vi "Check_Execution_Row.vi"(0 "Execution Row":T1 {"Row Duration (mins)" format="%#.1f"; "Row No" min=0; "Trace Gas Concentration (%)" min=0.0 format="%#.2f"; "Emission Rate (l/min)" format="%#.2f"; "Tunnel Speed" format="%#.2f"; "Start X" format="%#.2f"; "Start Y" format="%#.2f"; "Start Z" format="%#.2f"; "End X" format="%#.2f"; "End Y" format="%#.2f"; "End Z" format="%#.2f"; "Averaging time (min)" min=0.0 format="%#.2f"}, 3 "Synchronization Start No":i32=1 min=1 max=100, 4 "Row Index":i32, 5 "Max Tunnel Speed":dbl format="%.2f") -> (6 "Editted Row":bool, 7 "Execution Row Out":T1 {"Row Duration (mins)" format="%#.1f"; "Row No" min=0; "Trace Gas Concentration (%)" min=0.0 format="%#.2f"; "Emission Rate (l/min)" format="%#.2f"; "Tunnel Speed" format="%#.2f"; "Start X" format="%#.2f"; "Start Y" format="%#.2f"; "Start Z" format="%#.2f"; "End X" format="%#.2f"; "End Y" format="%#.2f"; "End Z" format="%#.2f"; "Averaging time (min)" min=0.0 format="%#.2f"}, 9 "Continue?":bool, 10 "Error Comments":string)   [LabVIEW 2012]
uses:
  Traverse_cluster.ctl
  Spacing.ctl
  Controls/Multi_run_mode.ctl
  Controls/User_Specific_mode.ctl
  Controls/Tunnel_Coordinates.ctl
  ADAM Client/Sub VIs/ADAM Controls/Channel_names.ctl
  Globals/Extra_Commands_Global.vi
  Globals/Constants_global.vi
  Globals/Trav_pos_global.vi
panel:
  out "Traverse line Out":T1 {"Row Duration (mins)" format="%#.1f"; "Row No" min=0; "Trace Gas Concentration (%)" min=0.0 format="%#.2f"; "Emission Rate (l/min)" format="%#.2f"; "Tunnel Speed" format="%#.2f"; "Start X" format="%#.2f"; "Start Y" format="%#.2f"; "Start Z" format="%#.2f"; "End X" format="%#.2f"; "End Y" format="%#.2f"; "End Z" format="%#.2f"; "Averaging time (min)" min=0.0 format="%#.2f"}
  out "Fixed Axis":bool[](array[boolean])
  out "Filenames":string[](array[string])
  out "Current Sync Number":i32
  out "Checks":string[](array[string])
  in  "Edit in Excel":bool
  in  "OK":bool
  # "X           Y            Z"
  # "Start"
  # "End"
  # "X           Y            Z"
  # "Start"
  # "End"
  # "X           Y            Z"
  # "Start"
  # "End"
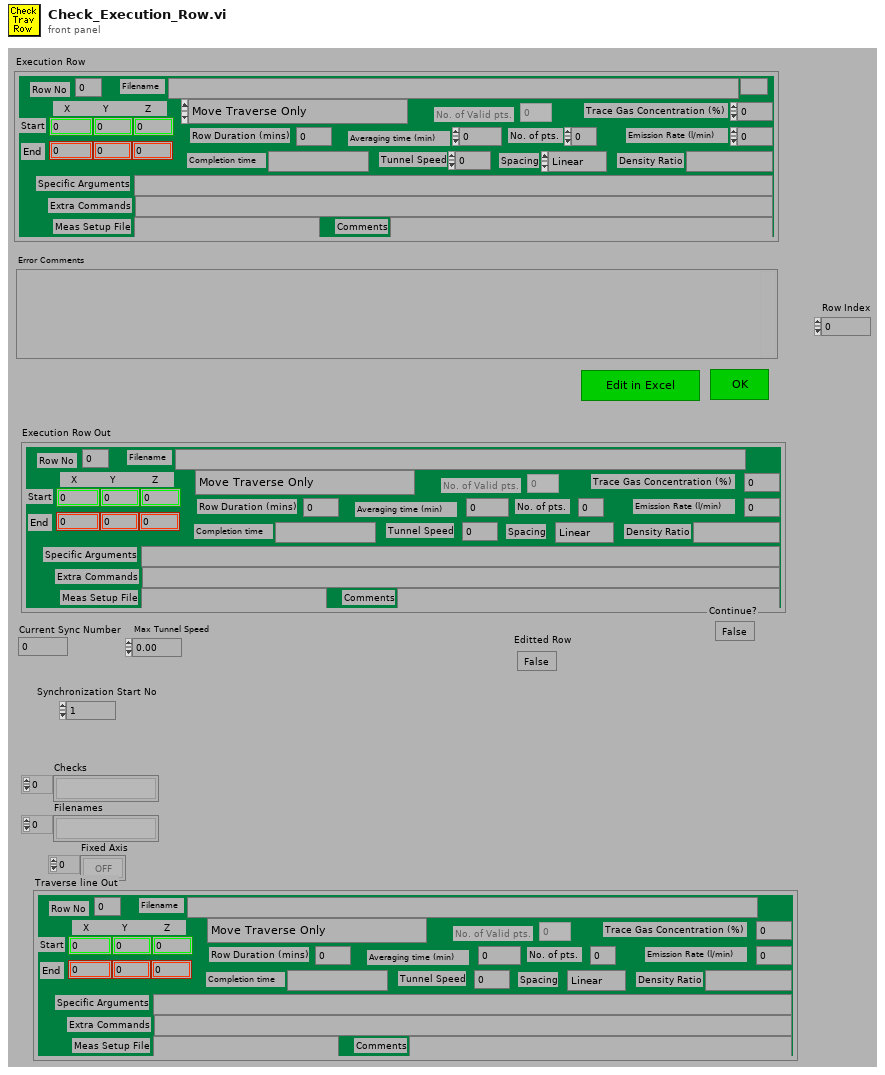
[diagram p1: front panel]
types:
  T1 = typedef "Traverse_cluster.ctl" = cluster{"Start X":dbl, "Start Y":dbl, "Start Z":dbl, "End X":dbl, "End Y":dbl, "End Z":dbl, "No. of pts.":i32, "Spacing":T2, "Filename":path, "Tunnel Speed":dbl, "Averaging time (min)":dbl, "Extra Commands":string, "Specific Arguments":string, "Emission Rate (l/min)":dbl, "Trace Gas Concentration (%)":dbl, "Density Ratio":string, "Comments":string, "Row No":i32, "Row Type Selector":T3, "Completion time":string, "Row Duration (mins)":dbl, "No. of Valid pts.":i32, "Meas Setup File":string}
  T2 = typedef "Spacing.ctl" = enum16{"Linear", "Log", "Gauss", "Specified", "N/A"}
  T3 = typedef "Multi_run_mode.ctl" = enum16{"Move Traverse Only", "Set Tunnel Speed Only", "Set Source Only", "Set Measurement Conditions", "Single Measurement", "Vertical Profile", "Lateral Profile", "Longitudinal Profile", "Explore Volume", "Multi-Axis Profile", "Auto Calibrate", "Meas Fast FID Bkgnd", "Check Beam Power", "Scanning Valve Measurement", "Run VI Named:", "Set ADAM Ch", "Wait (minutes)", "Send Message", "Synchronize With:", "Fall Back to this Row", "Turn Off Row Repeating", "Blank Row", "Traverse 3D Volume"}
  T4 = enum16{"All Channel Names", "Valid Channel Names"}
  T5 = typedef "User_Specific_mode.ctl" = enum16{"Check VI only", "Run VI"}
  T6 = typedef "Tunnel_Coordinates.ctl" = enum16{"Work in Tunnel Coordinates", "Work in Model Coordinates"}
  T7 = enum16{"Zero or one", "One", "Zero or more", "One or more"}
  T8 = typedef "Channel_names.ctl" = enum16{"Active Only", "Active + Off", "All Channels"}
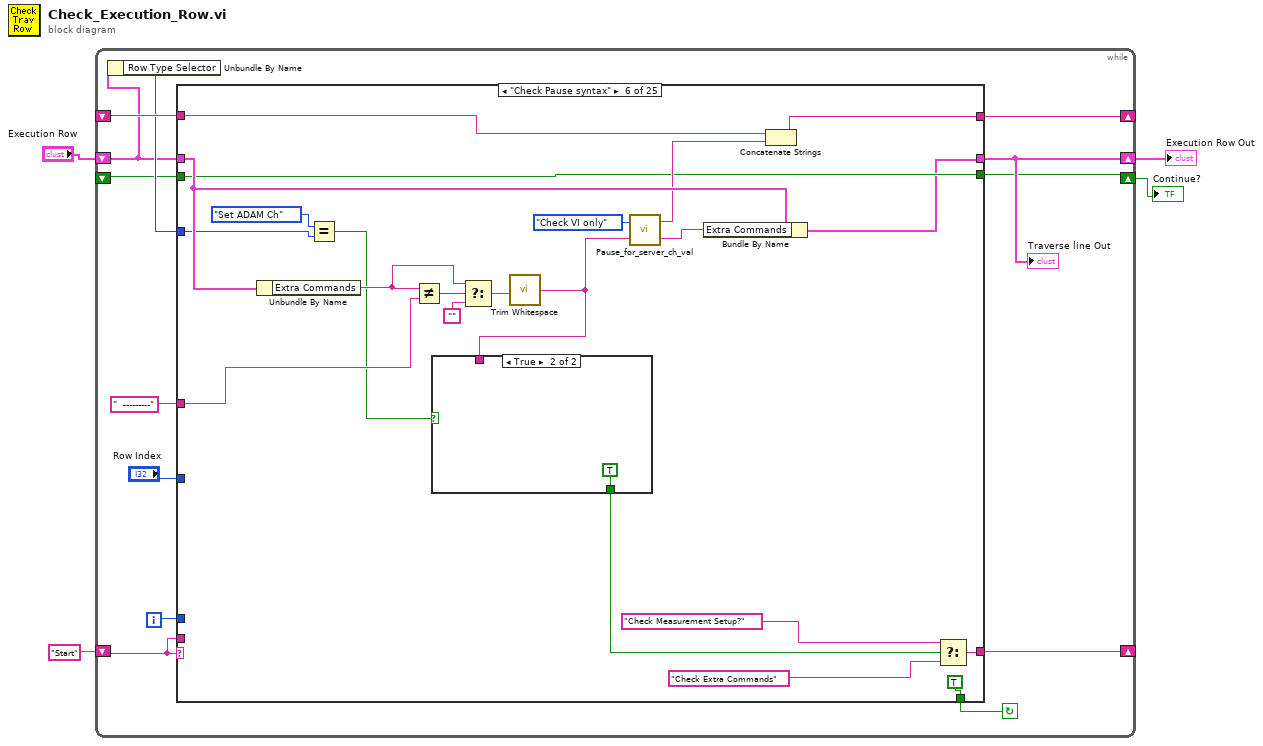
[diagram p0: block diagram]
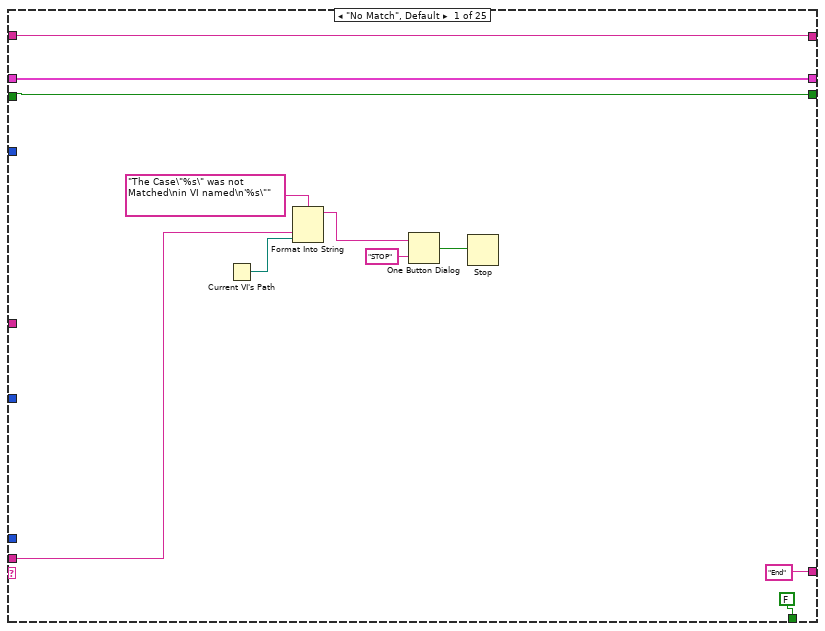
[diagram p2: hidden frame]
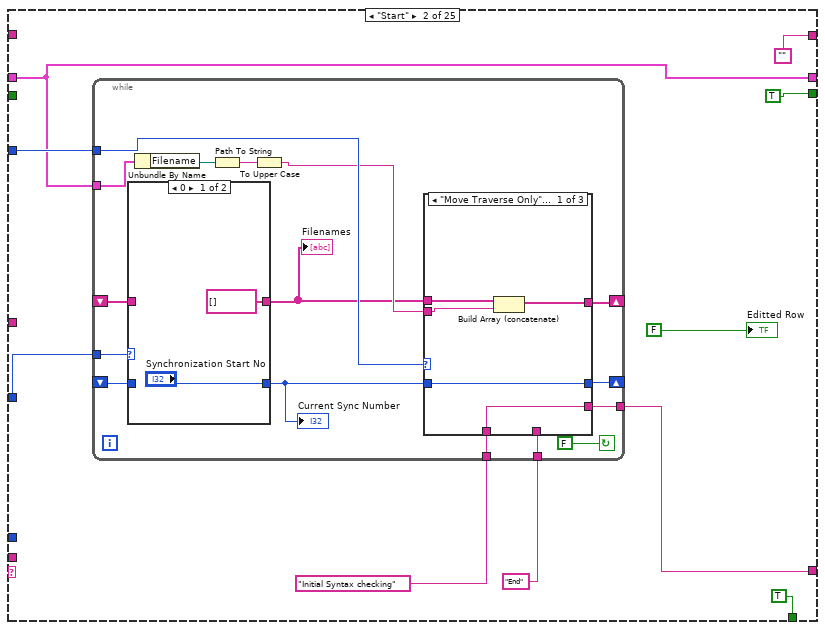
[diagram p3: hidden frame]
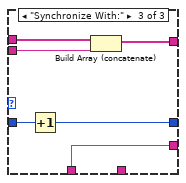
[diagram p6: hidden frame]
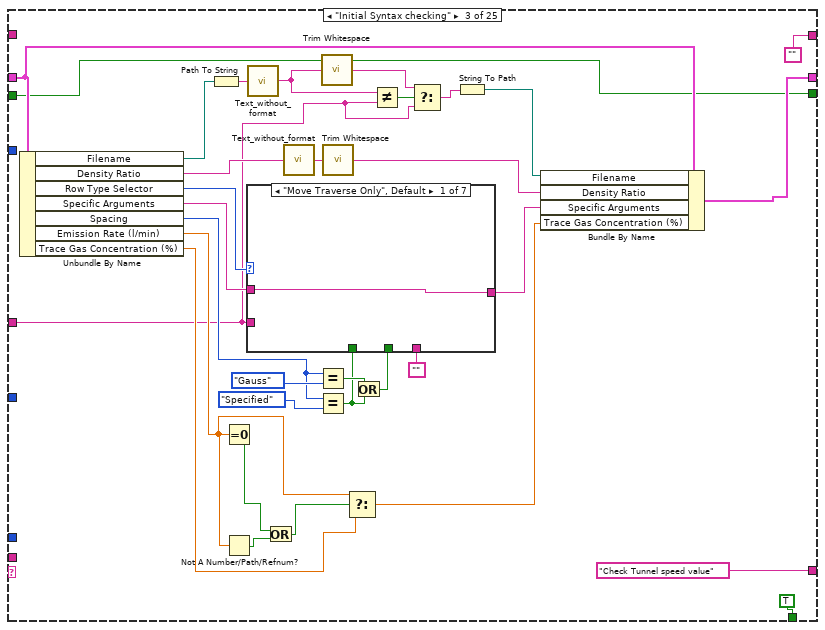
[diagram p7: hidden frame]
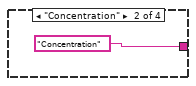
[diagram p9: hidden frame]
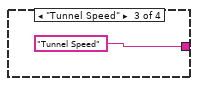
[diagram p10: hidden frame]
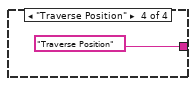
[diagram p11: hidden frame]
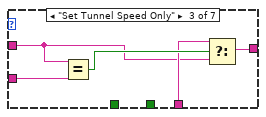
[diagram p12: hidden frame]
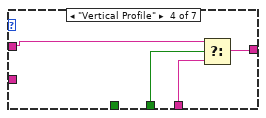
[diagram p13: hidden frame]
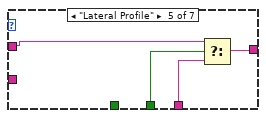
[diagram p14: hidden frame]
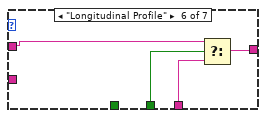
[diagram p15: hidden frame]
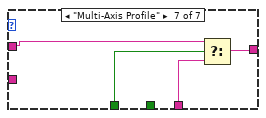
[diagram p16: hidden frame]
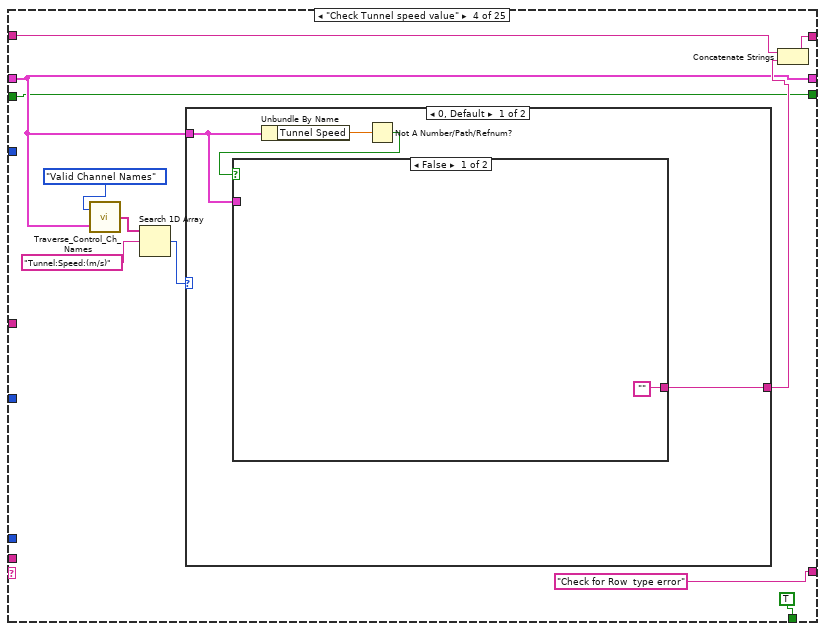
[diagram p17: hidden frame]
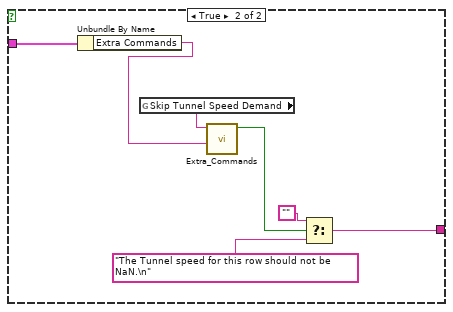
[diagram p18: hidden frame]
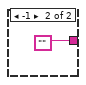
[diagram p19: hidden frame]
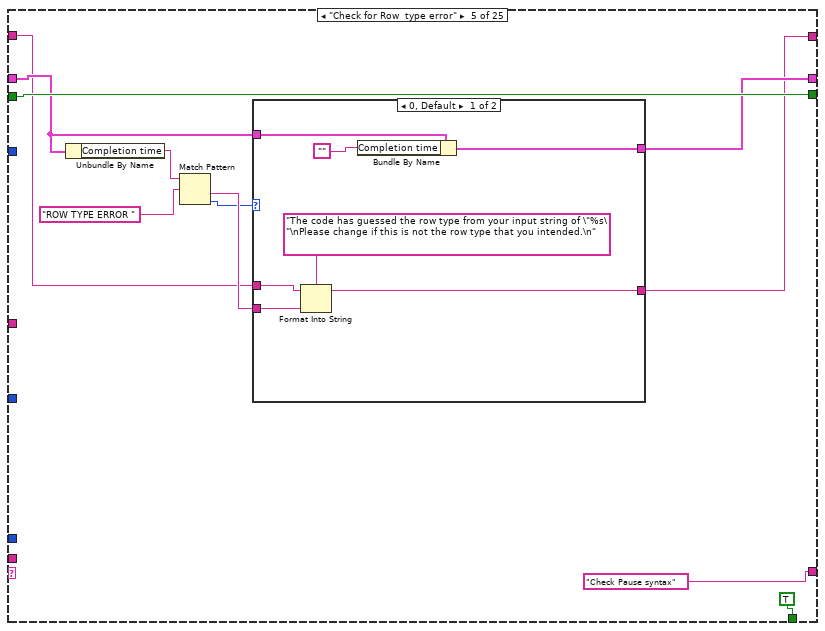
[diagram p20: hidden frame]
diagram:
  n1 = while {
    shift-left: _ -> [w16]
    shift-right: [w17] -> _
    shift-left: "Start" -> [w9]
    shift-right: [w14] -> _
    shift-right: [w8] -> w2
    shift-left: "Execution Row" -> [w5]
    shift-right: [w7] -> w1
    shift-left: _ -> [w6]
    i -> [w10]
    stop <- w15 continue-if-true
    n2 = Unbundle By Name(w5) -> ("Row Type Selector"=w12:T3)
    n3 = case shown="\"Check Pause syntax\"" w9 {
      tunnel: w5 -> [w22 w32 w100 w137 w161 w193 w211 w252 w282 w338 w371 w379 w418 w762 w862 w899 w927 w1012 w1044 w1054 w1123 _ w1162 w1169 w1179]
      tunnel: "  ---------" ("f") -> [_ _ w74 _ _ w197 _ _ _ _ _ _ _ _ _ _ _ _ _ _ _ _ _ _ _]
      tunnel: "Row Index" -> [_ w36 _ _ _ _ w208 _ _ _ _ _ w412 _ _ _ _ _ _ _ _ _ w1163 _ w1178]
      tunnel: [w21 "" "" w138 w158 w186 w219 w257 w287 w340 w375 w384 w422 w767 w872 w905 w950 w1010 w1048 w1055 w1129 w1140 w1164 w1174 w1181] -> w17
      tunnel: w12 -> [_ w35 _ _ _ w179 _ _ _ _ _ w382 w421 w763 w860 _ _ _ _ w1059 _ _ _ _ _]
      tunnel: w16 -> [w21 _ _ w139 w159 w188 w220 w258 w288 w340 w374 w385 w423 w767 w873 w906 w951 w1010 w1049 w1060 w1129 w1140 w1164 w1174 w1181]
      tunnel: [FALSE TRUE TRUE TRUE TRUE TRUE TRUE TRUE TRUE TRUE TRUE TRUE TRUE TRUE TRUE TRUE TRUE TRUE TRUE w1051 TRUE TRUE TRUE TRUE FALSE] -> w15
      tunnel: ["End" w33 "Check Tunnel speed value" ("f") "Check for Row  type error" ("f") "Check Pause syntax" ("f") w191 "Check Traverse Setup Name" ("f") "Check IF command" ("f") "Check Measurement Setup?" ("f") w342 "Check Maximum tunnel speed" ("f") "Row type specific check" ("f") w419 "Check for position NaNs" ("f") w863 "Check source details" ("t") "Check source details" ("f") w1007 "check entered filename etc" ("f") w1057 "What to do next?" ("f") w1138 "Initial Syntax checking" "End" "End"] -> w14
      tunnel: w10 -> [_ _ _ _ _ _ _ _ _ _ _ _ _ _ _ _ _ _ _ _ _ _ _ _ _]
      tunnel: w9 -> [w23 _ _ _ _ _ _ _ _ _ _ _ _ _ _ _ _ _ _ _ _ _ _ _ _]
      tunnel: [w22 w32 w77 w137 w162 w181 w210 w252 w282 w338 w370 w379 w413 w761 w862 w899 w926 w1011 w1044 w1053 w1123 w1131 w1165 w1169 w1177] -> w8
      tunnel: [w18 TRUE w75 w136 w168 w182 w212 w249 w279 w344 w372 w377 w415 w759 w861 w898 w924 w1015 w1042 w1051 w1122 w1130 w1159 w1168 w1175] -> w7
      tunnel: w6 -> [w18 _ w75 w136 w168 w182 w212 w249 w279 w344 w372 w377 w415 w759 w861 w898 w924 w1015 w1042 _ w1122 _ w1159 w1168 w1175]
      frame "No Match", Default {
        n4 = Current VI's Path() -> (path=w24:path)
        n5 = Format Into String(format string="The Case\"%s\" was not Matched\nin VI named\n'%s\"" ("Format String"), w23, w24) -> (resulting string=w27:string)  [unwired: 2 in, 1 out]
        n6 = One Button Dialog(message=w27, button name ("OK")="STOP") -> (true=w25:bool)
        n7 = Stop(stop? (T)=w25) -> ()
      }
      frame "Start" {
        n8 = while {
          tunnel: "End" -> [w40]
          tunnel: "Initial Syntax checking" -> [w41]
          tunnel: [w42] -> w33
          tunnel: w32 -> [w49]
          shift-left: _ -> [w48]
          shift-right: [w47] -> _
          tunnel: w35 -> [w53]
          shift-left: _ -> [w52]
          shift-right: [w51] -> _
          tunnel: w36 -> [w54]
          stop <- FALSE continue-if-true
          n9 = case shown="0" w54 {
            tunnel: ["Synchronization Start No" w58] -> w50
            tunnel: w52 -> [_ w58]
            tunnel: w48 -> [_ w57]
            tunnel: [string[] [] w57] -> w43
            frame 0 {
            }
            frame 1, Default {
            }
          }
          "Current Sync Number" <- w50
          "Filenames" <- w43
          n10 = Unbundle By Name(w49) -> ("Filename"=w46:path)
          n11 = Path To String(path=w46) -> (string=w45:string)
          n12 = To Upper Case(1:w45) -> (0:w44:string)
          n13 = case shown="\"Move Traverse Only\", Default" w53 {
            tunnel: w50 -> [w63 w66 w72]
            tunnel: [w63 w66 w71] -> w51
            tunnel: w44 -> [w61 _ w70]
            tunnel: w43 -> [w62 w65 w69]
            tunnel: [w60 w65 w68] -> w47
            tunnel: [w59 w64 w67] -> w42
            tunnel: w41 -> [w59 _ w67]
            tunnel: w40 -> [_ w64 _]
            frame "Move Traverse Only", Default {
              n14 = Build Array (concatenate)(w62, w61) -> (w60:string[])
            }
            frame "Blank Row" {
            }
            frame "Synchronize With:" {
              n15 = Increment(x=w72) -> (x+1=w71:i32)
              n16 = Build Array (concatenate)(w69, w70) -> (w68:string[])
            }
          }
        }
        "Editted Row" <- FALSE ("Editted Row")
      }
      frame "Initial Syntax checking" {
        n17 = Unbundle By Name(w100) -> ("Filename"=w73:path, "Density Ratio"=w79:string, "Row Type Selector"=w97:T3, "Specific Arguments"=w95:string, "Spacing"=w87:T2, "Emission Rate (l/min)"=w83:dbl, "Trace Gas Concentration (%)"=w93:dbl)
        n18 = Path To String(path=w73) -> (string=w81:string)
        n19 = Equal To 0?(x=w83) -> (x = 0?=w85:bool)
        n20 = Not A Number/Path/Refnum?(number/path/refnum=w83) -> (NaN/Path/Refnum?=w84:bool)
        n21 = call "Text_without_format.vi"("Input string"=w81) -> ("Output string"=w104:string)
        n22 = Or(x=w85, y=w84) -> (x .or. y?=w82:bool)
        n23 = call "Text_without_format.vi"("Input string"=w79) -> ("Output string"=w99:string)
        n24 = Equal?(x=w87, y=Spacing."Gauss" ("Spacing")) -> (x = y?=w89:bool)
        n25 = Equal?(x=w87, y=Spacing."Specified" ("Spacing")) -> (x = y?=w86:bool)
        n26 = call <vilib>:"Trim Whitespace.vi"("string"=w104) -> ("trimmed string"=w103:string)  [unwired: 1 in]
        n27 = call <vilib>:"Trim Whitespace.vi"("string"=w99) -> ("trimmed string"=w78:string)  [unwired: 1 in]
        n28 = Select(t=w83, s=w82, f=w93) -> (s? t:f=w92:dbl)
        n29 = Or(x=w89, y=w86) -> (x .or. y?=w88:bool)
        n30 = case shown="\"Move Traverse Only\", Default" w97 {
          tunnel: [w106 w108 w113 w119 w123 w127 w131] -> w96
          tunnel: w95 -> [w106 w107 w114 w121 w125 w129 w133]
          tunnel: "" -> [_ _ w115 w120 w124 w128 w132]
          tunnel: w88 -> [_ _ _ w118 w122 w126 _]
          tunnel: w86 -> [_ _ _ _ _ _ w130]
          tunnel: w74 -> [_ _ w117 _ _ _ _]
          frame "Move Traverse Only", Default {
          }
          frame "Auto Calibrate" {
            n31 = case shown="\"No Match\", Default" w107 {
              tunnel: [w109 "Concentration" "Tunnel Speed" "Traverse Position"] -> w108
              tunnel: w107 -> [w109 _ _ _]
              frame "No Match", Default {
              }
              frame "Concentration" {
              }
              frame "Tunnel Speed" {
              }
              frame "Traverse Position" {
              }
            }
          }
          frame "Set Tunnel Speed Only" {
            n32 = Equal?(x=w114, y=w117) -> (x = y?=w116:bool)
            n33 = Select(t=w115, s=w116, f=w114) -> (s? t:f=w113:string)
          }
          frame "Vertical Profile" {
            n34 = Select(t=w121, s=w118, f=w120) -> (s? t:f=w119:string)
          }
          frame "Lateral Profile" {
            n35 = Select(t=w125, s=w122, f=w124) -> (s? t:f=w123:string)
          }
          frame "Longitudinal Profile" {
            n36 = Select(t=w129, s=w126, f=w128) -> (s? t:f=w127:string)
          }
          frame "Multi-Axis Profile" {
            n37 = Select(t=w133, s=w130, f=w132) -> (s? t:f=w131:string)
          }
        }
        n38 = Not Equal?(x=w104, y=w74) -> (x != y?=w105:bool)
        n39 = Select(t=w103, s=w105, f=w74) -> (s? t:f=w102:string)
        n40 = String To Path(string=w102) -> (path=w80:path)
        n41 = Bundle By Name(cluster=w100, "Filename"=w80, "Density Ratio"=w78, "Specific Arguments"=w96, "Trace Gas Concentration (%)"=w92) -> (w77:T1)
      }
      frame "Check Tunnel speed value" {
        n42 = call "Traverse_Control_Ch_Names.vi"("Traverse line"=w137, "Mode"=T4."Valid Channel Names") -> ("Channel names"=w143:string[])
        n43 = Search 1D Array(1D array=w143, element="Tunnel:Speed:(m/s)" ("Label for value")) -> (index of element=w141:i32)  [unwired: 1 out]
        n44 = case shown="0, Default" w141 {
          tunnel: w137 -> [w146 _]
          tunnel: [w145 ""] -> w140
          frame 0, Default {
            n45 = Unbundle By Name(w146) -> ("Tunnel Speed"=w148:dbl)
            n46 = Not A Number/Path/Refnum?(number/path/refnum=w148) -> (NaN/Path/Refnum?=w147:bool)
            n47 = case shown="False" w147 {
              tunnel: w146 -> [_ w156]
              tunnel: ["" w150] -> w145
              frame False {
              }
              frame True {
                n48 = Unbundle By Name(w156) -> ("Extra Commands"=w154:string)
                n49 = global read "Extra_Commands_Global.vi" "Skip Tunnel Speed Demand"() -> (w155:string)
                n50 = call "Extra_Commands.vi"("String to Search"=w154, "Command"=w155) -> ("Command Found"=w153:bool)  [unwired: 1 in, 4 out]
                n51 = Select(t="", s=w153, f="The Tunnel speed for this row should not be NaN.\n") -> (s? t:f=w150:string)
              }
            }
          }
          frame -1 {
          }
        }
        n52 = Concatenate Strings(w139, w140) -> (w138:string)
      }
      frame "Check for Row  type error" {
        n53 = Unbundle By Name(w161) -> ("Completion time"=w164:string)
        n54 = Match Pattern(string=w164, regular expression="ROW TYPE ERROR " ("format string")) -> (after substring=w163:string, offset past match=w160:i32)  [unwired: 3 out]
        n55 = case shown="0, Default" w160 {
          tunnel: w163 -> [w175 _]
          tunnel: [w173 w177] -> w162
          tunnel: w161 -> [w172 w177]
          tunnel: [w170 w176] -> w158
          tunnel: w159 -> [w169 w176]
          frame 0, Default {
            n56 = Format Into String(format string="The code has guessed the row type from your input string of \"%s\"\nPlease change if this is not the row type that you intended.\n", initial string=w169, w175) -> (resulting string=w170:string)  [unwired: 1 in, 1 out]
            n57 = Bundle By Name(cluster=w172, "Completion time"="") -> (w173:T1)
          }
          frame -1 {
          }
        }
      }
      frame "Check Pause syntax" {
        n58 = Unbundle By Name(w193) -> ("Extra Commands"=w198:string)
        n59 = Equal?(x=Multi_run_mode."Set ADAM Ch" ("Row Type Selector"), y=w179) -> (x = y?=w178:bool)
        n60 = Not Equal?(x=w198, y=w197) -> (x != y?=w199:bool)
        n61 = Select(t=w198, s=w199, f="") -> (s? t:f=w195:string)
        n62 = call <vilib>:"Trim Whitespace.vi"("string"=w195) -> ("trimmed string"=w190:string)  [unwired: 1 in]
        n63 = case shown="True" w178 {
          tunnel: [w201 TRUE] -> w192
          tunnel: w190 -> [w200 _]
          frame False {
            n64 = Equal?(x=w200, y="") -> (x = y?=w201:bool)
          }
          frame True {
          }
        }
        n65 = call "Pause_for_server_ch_val.vi"("Extra command string"=w190, "Simulate/Run"=User_Specific_mode."Check VI only") -> ("Extra command string Out"=w189:string, "Error Comments"=w187:string)
        n66 = Bundle By Name(cluster=w193, "Extra Commands"=w189) -> (w181:T1)
        n67 = Concatenate Strings(w188, w187) -> (w186:string)
        n68 = Select(t="Check Measurement Setup?", s=w192, f="Check Extra Commands") -> (s? t:f=w191:string)
      }
      frame "Check Extra Commands" {
        n69 = Unbundle By Name(w211) -> ("Extra Commands"=w213:string)
        n70 = for {
          N: 3 -> [_]
          tunnel: w213 -> [w228]
          shift-right: [w224] -> w216
          shift-left: "" -> [w225]
          i -> [w230]
          n71 = case shown="0, Default" w230 {
            tunnel: [w233 w235 w237] -> w227
            tunnel: ["The Extra Command \"%s\" should have a numeric argument of (Centre; Intensity) eg 0 ; 0.85 for Gaussian spacing or (Offset) eg 300 for Log \n" ("Format String") "The Extra Command \"%s\" should have a numeric argument.\n" ("Format String") "The Extra Command \"%s\" should have a numeric argument.\n" ("Format String")] -> w222
            frame 0, Default {
              n72 = global read "Extra_Commands_Global.vi" "Point Spacing Parameters"() -> (w233:string)
            }
            frame 1 {
              n73 = global read "Extra_Commands_Global.vi" "Establish Exp Conditions (s)"() -> (w235:string)
            }
            frame 2 {
              n74 = global read "Extra_Commands_Global.vi" "Minutes Before Repeating Row"() -> (w237:string)
            }
          }
          n75 = call "Extra_Commands.vi"("String to Search"=w228, "Command"=w227) -> ("String Value"=w229:string, "Command Found"=w231:bool)  [unwired: 1 in, 3 out]
          n76 = case shown="True" w231 {
            tunnel: w229 -> [_ w246]
            tunnel: w227 -> [_ w244]
            tunnel: [w238 w241] -> w226
            tunnel: "" -> [w238 w240]
            tunnel: w222 -> [_ w239]
            frame False {
            }
            frame True {
              n77 = Decimal String To Number(string=w246) -> (offset past number=w245:i32)  [unwired: 3 out]
              n78 = Equal To 0?(x=w245) -> (x = 0?=w243:bool)
              n79 = Format Into String(format string=w239, w244) -> (resulting string=w242:string)  [unwired: 2 in, 1 out]
              n80 = Select(t=w242, s=w243, f=w240) -> (s? t:f=w241:string)
            }
          }
          n81 = Concatenate Strings(w226, w225) -> (w224:string)
        }
        n82 = call "Trav_Prog_Extra_Commands.vi"() -> ("Extra Commands Array"=w214:string[])  [unwired: 2 out]
        n83 = call "Valid_Extra_Command.vi"("Extra Commands string"=w213, "Valid Commands Array"=w214) -> ("Output String"=w218:string, "Extra Commands string Out"=w209:string)  [unwired: 3 out]
        n84 = Bundle By Name(cluster=w211, "Extra Commands"=w209) -> (w210:T1)
        n85 = call "Skip_If Sd_Error_Below.vi"("String to Search"=w209, "Simulate/Run"=User_Specific_mode."Check VI only", "Measurement setup Applied?"=FALSE, "Row Number"=w208) -> ("Error String"=w205:string)  [unwired: 1 in, 4 out]
        n86 = Concatenate Strings(w220, w218, w216, w205) -> (w219:string)
      }
      frame "Check Traverse Setup Name" {
        n87 = Unbundle By Name(w252) -> ("Extra Commands"=w248:string)
        n88 = global read "Extra_Commands_Global.vi" "!Traverse Setup"() -> (w255:string)
        n89 = call "Extra_Commands.vi"("String to Search"=w248, "Command"=w255) -> ("String Value"=w253:string, "Command Found"=w254:bool)  [unwired: 1 in, 3 out]
        n90 = case shown="True" w254 {
          tunnel: w253 -> [_ w265]
          tunnel: [w259 w262] -> w250
          tunnel: "" -> [w259 w261]
          frame False {
          }
          frame True {
            n91 = global read "Constants_global.vi" "Traverse folder"() -> (w260:path)
            n92 = List Folder(path=w260) -> (folder names=w263:string[])  [unwired: 1 in, 5 out]
            n93 = Search 1D Array(1D array=w263, element=w265) -> (index of element=w266:i32)  [unwired: 1 out]
            n94 = Greater Or Equal To 0?(x=w266) -> (x >= 0?=w264:bool)
            n95 = case shown="False" w264 {
              tunnel: w265 -> [w271 _]
              tunnel: w263 -> [w268 _]
              tunnel: [w267 w276] -> w262
              tunnel: w261 -> [_ w276]
              frame False {
                n96 = Format Into String(format string="%s is not a valid Travese setup. Valid option are:", w271) -> (resulting string=w269:string)  [unwired: 2 in, 1 out]
                n97 = for {
                  shift-right: [w273] -> w267
                  shift-left: w269 -> [w274]
                  tunnel: w268 -> [w275] mode=indexing
                  w272 = "  " ("Substring")
                  n98 = Concatenate Strings(w274, w272, w275, w272) -> (w273:string)
                }
              }
              frame True {
              }
            }
          }
        }
        n99 = Concatenate Strings(w258, w250) -> (w257:string)
      }
      frame "Check IF command" {
        n100 = Unbundle By Name(w282) -> ("Extra Commands"=w278:string)
        n101 = global read "Extra_Commands_Global.vi" "If Command"() -> (w285:string)
        n102 = call "Extra_Commands.vi"("String to Search"=w278, "Command"=w285) -> ("String Value"=w283:string, "Command Found"=w284:bool)  [unwired: 1 in, 3 out]
        n103 = case shown="True" w284 {
          tunnel: w283 -> [_ w294]
          tunnel: [w289 w293] -> w280
          tunnel: "" -> [w289 w291]
          frame False {
          }
          frame True {
            n104 = call "Get_array_values_fr_String.vi"("String Value"=w294) -> ("Numeric Array"=w290:dbl[], "String array"=w292:string[])
            n105 = Index Array(array=w292, index=0 ("Index")) -> (element=w295:string)
            n106 = case shown="\"Global Value Between\"" w295 {
              tunnel: w294 -> [w300 _ _ _]
              tunnel: [w299 w325 w326 "The !If  command has not been recognised.\nExtra command Example:\n!IF = Time Between;10:45;and;14:00;Execute Row (or) Skip Row\n\n!IF = ADAM Channel Between;Channel Name; 0.5;1.0\n\n!IF = Global Value Between; 0.5;1.0" ("Error Comments")] -> w293
              tunnel: w292 -> [_ w316 w334 _]
              tunnel: w291 -> [_ w309 w327 _]
              tunnel: w290 -> [_ _ _ _]
              frame "Time Between" {
                n107 = Get Date/Time In Seconds() -> (seconds since 1Jan1904=w297:timestamp)
                n108 = To Double Precision Float(number=w297) -> (double precision float=w298:dbl)
                n109 = call "If_Time_arguments.vi"("seconds since 1Jan1904"=w298, "String Value"=w300) -> ("Error Comments"=w299:string)  [unwired: 2 out]
              }
              frame "ADAM Channel Between" {
                n110 = Index Array(array=w316, index=1 ("Index")) -> (element=w319:string)
                n111 = Index Array(array=w316, index=2 ("Index")) -> (element=w315:string)
                n112 = Index Array(array=w316, index=3 ("Index")) -> (element=w314:string)
                n113 = Build Array(w319) -> (w321:string[])
                n114 = Decimal Digit?(1:w315) -> (0:w312:bool)
                n115 = Decimal Digit?(1:w314) -> (0:w313:bool)
                n116 = call "Get_Current_Scan_client.vi"("ADAM Ch Names"=w321) -> ("Numerical Values"=w323:dbl[])  [unwired: 3 out]
                n117 = And(x=w312, y=w313) -> (x .and. y?=w311:bool)
                n118 = Index Array(array=w323, index=0 ("Index")) -> (element=w324:dbl)
                n119 = Select(t=w309, s=w311, f="you must give two limits\n") -> (s? t:f=w305:string)
                n120 = Not A Number/Path/Refnum?(number/path/refnum=w324) -> (NaN/Path/Refnum?=w308:bool)
                n121 = Select(t="Invalid ADAM Channel Name\n", s=w308, f=w309) -> (s? t:f=w306:string)
                n122 = Concatenate Strings(w306, w305) -> (w303:string)
                n123 = Concatenate Strings(w303, "Extra command Example:\n!IF = ADAM Channel Between;Channel Name; 0.5;1.0") -> (w302:string)
                n124 = Empty String/Path?(string/path=w303) -> (empty?=w304:bool)
                n125 = Select(t=w309, s=w304, f=w302) -> (s? t:f=w325:string)
              }
              frame "Global Value Between" {
                n126 = Index Array(array=w334, index=1 ("Index")) -> (element=w333:string)
                n127 = Index Array(array=w334, index=2 ("Index")) -> (element=w332:string)
                n128 = Decimal Digit?(1:w333) -> (0:w330:bool)
                n129 = Decimal Digit?(1:w332) -> (0:w331:bool)
                n130 = And(x=w330, y=w331) -> (x .and. y?=w329:bool)
                n131 = Select(t=w327, s=w329, f="The Extra command IF statement must have two numerical values for the limits\n\nExtra command Example:\n!IF = Global Value Between; 0.5;1.0") -> (s? t:f=w326:string)
              }
              frame "No Match", Default {
              }
            }
          }
        }
        n132 = Concatenate Strings(w288, w280) -> (w287:string)
      }
      frame "Check Measurement Setup?" {
        n133 = Unbundle By Name(w338) -> ("Row Type Selector"=w343:T3, "Specific Arguments"=w341:string)
        n134 = case shown="\"Traverse 3D Volume\"" w343 {
          tunnel: ["Check Measurement Setup" ("t") "Check Measurement Setup" ("t") "Check Measurement Setup" ("t") "Check Measurement Setup" ("t") "Check Measurement Setup" ("t") "Check Measurement Setup" ("t") "Check Measurement Setup" ("t") "Check Measurement Setup" ("t") "Check Measurement Setup" ("t") "Check Measurement Setup" ("t") "Check Measurement Setup" ("t") w357 w366] -> w342
          tunnel: w341 -> [_ _ _ _ _ _ _ _ _ _ _ w364 _]
          tunnel: "Check Maximum tunnel speed" ("f") -> [_ _ _ _ _ _ _ _ _ _ _ w358 w366]
          tunnel: w338 -> [_ _ _ _ _ _ _ _ _ _ _ w361 _]
          frame "Lateral Profile" {
          }
          frame "Traverse 3D Volume" {
          }
          frame "Longitudinal Profile" {
          }
          frame "Explore Volume" {
          }
          frame "Multi-Axis Profile" {
          }
          frame "Vertical Profile" {
          }
          frame "Single Measurement" {
          }
          frame "Scanning Valve Measurement" {
          }
          frame "Auto Calibrate" {
          }
          frame "Meas Fast FID Bkgnd" {
          }
          frame "Check Beam Power" {
          }
          frame "Run VI Named:" {
            n135 = Match Pattern(string=w364, regular expression=";") -> (before substring=w363:string)  [unwired: 4 out]
            n136 = call <vilib>:"Trim Whitespace.vi"("string"=w363) -> ("trimmed string"=w362:string)  [unwired: 1 in]
            n137 = call "Run_VI_Named_specific.vi"("Run VI Named String"=w362, "Multi Run Row"=w361) -> ("Check Meas Setup?"=w360:bool)  [unwired: 9 out]
            n138 = Select(t="Check Measurement Setup", s=w360, f=w358) -> (s? t:f=w357:string)
          }
          frame "Set Tunnel Speed Only", Default {
          }
        }
      }
      frame "Check Measurement Setup" {
        n139 = Unbundle By Name(w371) -> ("Meas Setup File"=w369:string)
        n140 = call "Check_Measurement_Setups.vi"("Measurement Setup String"=w369) -> ("Measurement Setup String Out"=w368:string, "Error Comments"=w367:string)
        n141 = Bundle By Name(cluster=w371, "Meas Setup File"=w368) -> (w370:T1)
        n142 = Concatenate Strings(w374, w367) -> (w375:string)
      }
      frame "Check Maximum tunnel speed" {
        n143 = case shown="\"Set Tunnel Speed Only\", Default" w382 {
          tunnel: w379 -> [w404 _]
          tunnel: [w395 FALSE] -> w381
          tunnel: [w394 0.0] -> w380
          frame "Auto Calibrate" {
            n144 = Unbundle By Name(w404) -> ("Specific Arguments"=w403:string)
            n145 = call "Get_array_values_fr_String.vi"("String Value"=w403) -> ("Numeric Array"=w397:dbl[], "String array"=w402:string[])
            n146 = Index Array(array=w402, index=0 ("Index")) -> (element=w400:string)
            n147 = Equal?(x=w400, y="Tunnel Speed" ("Output Array")) -> (x = y?=w395:bool)
            n148 = Array Subset(array=w397, index=1 ("Array Index")) -> (w396:dbl[])  [unwired: 1 in]
            n149 = Array Max & Min(array=w396) -> (max value=w394:dbl)  [unwired: 3 out]
          }
          frame "Set Tunnel Speed Only", Default {
          }
        }
        n150 = case shown="False" w381 {
          tunnel: [w392 w393] -> w389
          tunnel: w379 -> [w391 _]
          tunnel: w380 -> [_ w393]
          frame False {
            n151 = Unbundle By Name(w391) -> ("Tunnel Speed"=w392:dbl)
          }
          frame True {
          }
        }
        n152 = Greater?(x=w389, y="Max Tunnel Speed") -> (0:w387:bool)
        n153 = Not A Number/Path/Refnum?(number/path/refnum=w389) -> (NaN/Path/Refnum?=w388:bool)
        n154 = Compound Arithmetic op=AND(invert w388, w387) -> (w386:bool)
        n155 = case shown="False" w386 {
          tunnel: w385 -> [w407 w409]
          tunnel: [w407 w408] -> w384
          tunnel: "Max Tunnel Speed" -> [_ w411]
          frame False {
          }
          frame True {
            n156 = Format Into String(format string="The maximum allowable tunnel speed is %.2f m/s.\n" ("Format String"), initial string=w409, w411) -> (resulting string=w408:string)  [unwired: 1 in, 1 out]
          }
        }
      }
      frame "Row type specific check" {
        n157 = case shown="\"Set ADAM Ch\"" w421 {
          tunnel: w418 -> [w432 w441 w445 w449 w454 w459 w466 w473 w484 w492 w506 w510 w587 w594 w615 w642 w690 w718 w723 w727 w739 w743 w749]
          tunnel: [string[] [] string[] [] string[] [] string[] [] w455 w462 w469 w476 w489 w497 w507 w532 w589 string[] [] w632 string[] [] w685 string[] [] string[] [] string[] [] string[] [] string[] [] string[] []] -> w420
          tunnel: [w426 "" "" "" "" "" "" "" w485 w494 "" w546 w583 w593 w627 w636 w701 w720 "" w729 "" "" w751] -> w424
          tunnel: [w435 w442 w446 w450 w453 w460 w467 w474 w483 w493 w505 w531 w577 w592 w626 w645 w686 "check entered filename etc" "check entered filename etc" "check entered filename etc" "check entered filename etc" "check entered filename etc" "check entered filename etc"] -> w419
          tunnel: "Check source details" -> [_ w442 w446 _ _ _ _ _ _ _ w505 _ w577 w592 w626 w644 w687 _ _ _ _ _ _]
          tunnel: "Sort out start and end positions" -> [_ _ _ _ _ w460 w467 w474 _ w493 _ w529 _ _ _ _ _ _ _ _ _ _ _]
          tunnel: "Check for Start NaNs" -> [w435 _ _ w450 w453 _ _ _ w483 _ _ w530 _ _ _ _ _ _ _ _ _ _ _]
          tunnel: [w431 w441 w445 w449 w454 w459 w466 w473 w484 w492 w506 w511 w587 w602 w615 w641 w690 w718 w723 w727 w739 w743 w747] -> w413
          tunnel: w412 -> [_ _ _ _ _ _ _ _ _ _ _ _ _ _ _ w647 _ _ _ _ _ _ _]
          frame "Move Traverse Only" {
            n158 = Unbundle By Name(w432) -> ("Specific Arguments"=w433:string)
            n159 = call <vilib>:"Trim Whitespace.vi"("string"=w433) -> ("trimmed string"=w427:string)  [unwired: 1 in]
            n160 = Equal?(x=w427, y="No Backlash") -> (x = y?=w430:bool)
            n161 = Empty String/Path?(string/path=w427) -> (empty?=w429:bool)
            n162 = Or(x=w429, y=w430) -> (x .or. y?=w428:bool)
            n163 = case shown="True" w428 {
              tunnel: w427 -> [w438 _]
              tunnel: [w437 ""] -> w426
              frame False {
                n164 = Format Into String(format string="\"%s\" is an Incorrect Specific Argument. It should either be left blank or say \"No Backlash\"\n", w438) -> (resulting string=w437:string)  [unwired: 2 in, 1 out]
              }
              frame True {
              }
            }
            n165 = Bundle By Name(cluster=w432, "Specific Arguments"=w427) -> (w431:T1)
          }
          frame "Set Tunnel Speed Only" {
          }
          frame "Set Source Only" {
          }
          frame "Set Measurement Conditions" {
          }
          frame "Single Measurement" {
            n166 = Build Array("Averaging:Time:(mins)" ("Label for value"), "Filename:HD:Users" ("Label for value")) -> (w455:string[])
          }
          frame "Vertical Profile" {
            n167 = Build Array("Number:Of:Points" ("Label for value"), "Averaging:Time:(mins)" ("Label for value"), "Filename:HD:Users" ("Label for value")) -> (w462:string[])
          }
          frame "Lateral Profile" {
            n168 = Build Array("Number:Of:Points" ("Label for value"), "Averaging:Time:(mins)" ("Label for value"), "Filename:HD:Users" ("Label for value")) -> (w469:string[])
          }
          frame "Longitudinal Profile" {
            n169 = Build Array("Number:Of:Points" ("Label for value"), "Averaging:Time:(mins)" ("Label for value"), "Filename:HD:Users" ("Label for value")) -> (w476:string[])
          }
          frame "Explore Volume" {
            n170 = Unbundle By Name(w484) -> ("Specific Arguments"=w482:string)
            n171 = Build Array("Averaging:Time:(mins)" ("Label for value"), "Filename:HD:Users" ("Label for value")) -> (w489:string[])
            n172 = Fract/Exp String To Number(string=w482) -> (number=w481:dbl)  [unwired: 4 out]
            n173 = Greater Than 0?(x=w481) -> (x > 0?=w480:bool)
            n174 = Format Into String(format string="\"%s\" is an Incorrect Specific Argument. Please enter the radius of the volume in mm.\n", w482) -> (resulting string=w486:string)  [unwired: 2 in, 1 out]
            n175 = Select(t="", s=w480, f=w486) -> (s? t:f=w485:string)
          }
          frame "Multi-Axis Profile" {
            n176 = Unbundle By Name(w492) -> ("Spacing"=w495:T2)
            n177 = case shown="\"Gauss\"" w495 {
              tunnel: ["" "You are not allowed to specify gaussian spacing for a Multi-Axis profile.\n" "You are not allowed to specify Log spacing for a Multi-Axis profile.\n" "\"N/A\" is not a valid point spacing.\n"] -> w494
              frame "Linear", Default {
              }
              frame "Gauss" {
              }
              frame "Log" {
              }
              frame "N/A" {
              }
            }
            n178 = Build Array("Number:Of:Points" ("Label for value"), "Averaging:Time:(mins)" ("Label for value"), "Filename:HD:Users" ("Label for value")) -> (w497:string[])
          }
          frame "Traverse 3D Volume" {
            n179 = Build Array("Averaging:Time:(mins)" ("Label for value"), "Filename:HD:Users" ("Label for value")) -> (w507:string[])
          }
          frame "Auto Calibrate" {
            n180 = Unbundle By Name(w510) -> ("Filename"=w514:path, "Specific Arguments"=w545:string)
            n181 = call "Get_array_values_fr_String.vi"("String Value"=w545) -> ("Numeric Array"=w541:dbl[], "String array"=w528:string[])
            n182 = global read "Trav_pos_global.vi" "Work in Tunnel Coordinates?"() -> (w524:T6)
            n183 = Index Array(array=w528, index=0 ("Index")) -> (element=w527:string)
            n184 = Build Array("Tunnel Speed", "Traverse Position", "Concentration") -> (w526:string[])
            n185 = Build Array("Averaging:Time:(mins)" ("Label for value")) -> (w532:string[])
            n186 = Array Size(array=w541) -> (size(s)=w540:i32)
            n187 = call "Current_Filepath.vi"("Filename in"=w514, "Data Type"="Calibrations") -> ("Filename Out"=w512:path)  [unwired: 1 out]
            n188 = Equal?(x=w524, y=Tunnel_Coordinates."Work in Model Coordinates" ("Work in Tunnel Coordinates?")) -> (x = y?=w518:bool)
            n189 = Search 1D Array(1D array=w526, element=w527) -> (index of element=w519:i32)  [unwired: 1 out]
            n190 = Equal?(x=2, y=w519) -> (x = y?=w521:bool)
            n191 = case shown="1" w519 {
              tunnel: [w575 w576] -> w531
              tunnel: w530 -> [w575 _]
              tunnel: w529 -> [_ w576]
              frame 0, Default {
              }
              frame 1 {
              }
            }
            n192 = Less?(x=w540, y=3) -> (x < y?=w536:bool)
            n193 = Equal To 0?(x=w519) -> (x = 0?=w537:bool)
            n194 = And(x=w518, y=w521) -> (x .and. y?=w520:bool)
            n195 = Greater Or Equal To 0?(x=w519) -> (x >= 0?=w517:bool)
            n196 = Compound Arithmetic op=AND(w536, w537) -> (w535:bool)
            n197 = case shown="True" w520 {
              tunnel: [w562 w567] -> w513
              tunnel: w510 -> [w562 w563]
              frame False {
              }
              frame True {
                n198 = Unbundle By Name(w563) -> ("Extra Commands"=w564:string)
                n199 = global read "Extra_Commands_Global.vi" "Work in Tunnel Coordinates"() -> (w565:string)
                n200 = call "Extra_Commands.vi"("String to Search"=w564, "Command"=w565) -> ("Command Found"=w566:bool)  [unwired: 1 in, 4 out]
                n201 = case shown="False" w566 {
                  tunnel: [w573 w574] -> w567
                  tunnel: w565 -> [w572 _]
                  tunnel: w564 -> [w571 _]
                  tunnel: w563 -> [w569 w574]
                  frame False {
                    n202 = Concatenate Strings(w572, "  " ("string"), w571) -> (w570:string)
                    n203 = Bundle By Name(cluster=w569, "Extra Commands"=w570) -> (w573:T1)
                  }
                  frame True {
                  }
                }
              }
            }
            n204 = Select(t="You need to enter the desired tunnel speeds in the \"Specfic Arguments\" Box   eg.  Tunnel Speed;1;2;3;4\n", s=w535, f="") -> (s? t:f=w533:string)
            n205 = call "Does_file_exist_(simple).vi"("Pathname"=w512) -> ("exists?"=w551:bool)
            n206 = case shown="False" w517 {
              tunnel: w526 -> [w553 _]
              tunnel: [w552 ""] -> w516
              frame False {
                n207 = for {
                  shift-right: [w558] -> w555
                  shift-left: "Incorrect Specific Argument. The options are: " -> [w559]
                  tunnel: w553 -> [w560] mode=indexing
                  w557 = "  " ("Substring")
                  n208 = Concatenate Strings(w559, w557, w560, w557) -> (w558:string)
                }
                n209 = Concatenate Strings(w555, "\r\n") -> (w552:string)
              }
              frame True {
              }
            }
            n210 = Select(t="", s=w551, f="The calibration file cannot be found.\n") -> (s? t:f=w547:string)
            n211 = Bundle By Name(cluster=w513, "Filename"=w512) -> (w511:T1)
            n212 = Concatenate Strings(w547, w533, w516) -> (w546:string)
          }
          frame "Meas Fast FID Bkgnd" {
            n213 = Unbundle By Name(w587) -> ("Specific Arguments"=w582:string)
            n214 = call "Get_array_values_fr_String.vi"("String Value"=w582) -> ("String array"=w581:string[])  [unwired: 1 out]
            n215 = Index Array(array=w581, index=0) -> (element=w579:string)
            n216 = Empty String/Path?(string/path=w579) -> (empty?=w585:bool)
            n217 = Build Array("Averaging:Time:(mins)" ("Label for value")) -> (w589:string[])
            n218 = Equal?(x=w579, y="Use Source Divertor Valve") -> (x = y?=w578:bool)
            n219 = Or(x=w585, y=w578) -> (x .or. y?=w584:bool)
            n220 = case shown="False" w584 {
              tunnel: ["Specific Argument should either be blank or\nUse Source Divertor Valve ; (wait time in seconds optional)" ""] -> w583
              frame False {
              }
              frame True {
              }
            }
          }
          frame "Check Beam Power" {
            n221 = Unbundle By Name(w594) -> ("Extra Commands"=w596:string, "Start X"=w601:dbl, "Start Y"=w599:dbl, "Start Z"=w600:dbl)
            n222 = global read "Extra_Commands_Global.vi" "Skip Traverse Position Demand"() -> (w597:string)
            n223 = call "Extra_Commands.vi"("String to Search"=w596, "Command"=w597) -> ("Command Found"=w595:bool)  [unwired: 1 in, 4 out]
            n224 = case shown="False" w595 {
              tunnel: w601 -> [w613 _]
              tunnel: w600 -> [w612 _]
              tunnel: w599 -> [w611 _]
              tunnel: "" -> [w608 w614]
              tunnel: [w607 w614] -> w593
              frame False {
                n225 = Build Array(w613, w611, w612) -> (w610:dbl[])
                n226 = Not A Number/Path/Refnum?(number/path/refnum=w610) -> (NaN/Path/Refnum?=w609:bool[])
                n227 = Or Array Elements(Boolean array=w609) -> (logical OR=w606:bool)
                n228 = Select(t="The start position is where the datum velocity measurement will be made. This should not contain NaNs.\n" ("f"), s=w606, f=w608) -> (s? t:f=w607:string)
              }
              frame True {
              }
            }
            n229 = Bundle By Name(cluster=w594, "Comments"="Start Position is the location of Datum Velocity Measurement") -> (w602:T1)
          }
          frame "Scanning Valve Measurement" {
            w628 = ext -0.5  # lo
            w629 = ext 47.5  # hi
            n230 = Unbundle By Name(w615) -> ("Specific Arguments"=w625:string)
            n231 = call "Get_array_values_fr_String.vi"("String Value"=w625) -> ("Numeric Array"=w624:dbl[], "String array"=w620:string[])
            n232 = Build Array("Averaging:Time:(mins)" ("Label for value"), "Filename:HD:Users" ("Label for value")) -> (w632:string[])
            n233 = Index Array(array=w620, index=0) -> (element=w619:string)
            n234 = Empty String/Path?(string/path=w619) -> (empty?=w617:bool)
            n235 = Index Array(array=w624, index=0) -> (element=w622:dbl)
            n236 = In Range and Coerce(upper limit=w629, x=w622, lower limit=w628) -> (In Range?=w618:bool)  [unwired: 1 out]
            n237 = Compound Arithmetic op=AND(invert w617, w618) -> (w616:bool)
            n238 = Select(t="", s=w616, f="Enter the scanning valve port number between 0 and 47 in the specific arguments box.\n") -> (s? t:f=w627:string)
          }
          frame "Set ADAM Ch" {
            n239 = while {
              shift-right: [w680] -> w649
              shift-left: _ -> [w673]
              shift-right: [w679] -> _
              shift-left: _ -> [w678]
              tunnel: w647 -> [w679]
              stop <- TRUE stop-if-true
              n240 = Array Size(array=w673) -> (size(s)=w677:i32)
              n241 = Less?(x=w679, y=w678) -> (x < y?=w675:bool)
              n242 = Equal To 0?(x=w677) -> (x = 0?=w676:bool)
              n243 = Or(x=w676, y=w675) -> (x .or. y?=w674:bool)
              n244 = case shown="True" w674 {
                tunnel: [w681 w682] -> w680
                tunnel: w673 -> [w681 _]
                frame False {
                }
                frame True {
                  n245 = call "Get_ADAM_Ch_names_client.vi"("Channel names set"=Channel_names."Active + Off") -> ("Ch names"=w682:string[])
                }
              }
            }
            n246 = Unbundle By Name(w642) -> ("Specific Arguments"=w653:string, "Extra Commands"=w635:string)
            n247 = call "Get_array_values_fr_String.vi"("String Value"=w653) -> ("String array"=w640:string[])  [unwired: 1 out]
            n248 = Index Array(array=w640, index=0) -> (element=w648:string)
            n249 = Empty String/Path?(string/path=w635) -> (empty?=w638:bool)
            n250 = Search 1D Array(1D array=w649, element=w648) -> (index of element=w651:i32)  [unwired: 1 out]
            n251 = Greater Or Equal To 0?(x=w651) -> (x >= 0?=w650:bool)
            n252 = Select(t="You have not specified a Value to Set the ADAM channel to.\nPlease give a value in the Extra Commands string", s=w638, f="") -> (s? t:f=w636:string)
            n253 = case shown="True" w650 {
              tunnel: w649 -> [w667 _]
              tunnel: w648 -> [w665 w668]
              tunnel: w647 -> [w663 _]
              tunnel: [w661 FALSE ("Cancel")] -> w646
              tunnel: w642 -> [w657 w670]
              tunnel: [w656 w669] -> w641
              tunnel: w635 -> [_ _]
              frame False {
                n254 = Build Array(w665) -> (w664:string[])
                n255 = Format Into String(format string="Please Select the ADAM Channel that you want to set in row %d", w663) -> (resulting string=w662:string)  [unwired: 2 in, 1 out]
                n256 = call "Select_Strings.vi"("Available Ch names"=w667, "Message"=w662, "Selector mode"=T7."One", "Desired Ch names (in)"=w664) -> ("Cancel"=w661:bool, "Selected Channel Names"=w659:string[])  [unwired: 3 out]
                n257 = Index Array(array=w659, index=0) -> (element=w655:string)
                n258 = Bundle By Name(cluster=w657, "Specific Arguments"=w655) -> (w656:T1)
              }
              frame True {
                n259 = Bundle By Name(cluster=w670, "Specific Arguments"=w668) -> (w669:T1)
              }
            }
            n260 = Select(t="Close Front Panel", s=w646, f=w644) -> (s? t:f=w645:string)
          }
          frame "Run VI Named:" {
            w695 = "Run_VI_Named_specific.vi"
            n261 = Unbundle By Name(w690) -> ("Specific Arguments"=w698:string)
            n262 = global read "Constants_global.vi" "Run VI Folder"() -> (w696:path)
            n263 = Match Pattern(string=w698, regular expression=";") -> (before substring=w699:string)  [unwired: 4 out]
            n264 = call <vilib>:"Trim Whitespace.vi"("string"=w699) -> ("trimmed string"=w691:string)  [unwired: 1 in]
            n265 = call "Run_VI_Named_specific.vi"("Run VI Named String"=w691, "Multi Run Row"=w690) -> ("Checks"=w685:string[], "Error String"=w684:string, "Check for start NaNs?"=w689:bool)  [unwired: 7 out]
            n266 = Select(t="Check for Start NaNs" ("Label for value"), s=w689, f=w687) -> (s? t:f=w686:string)
            n267 = Build Path(base path=w696, name or relative path=w691) -> (appended path=w702:path)
            n268 = Not Equal?(x=w691, y=w695) -> (x != y?=w694:bool)
            n269 = call "Does_file_exist_(simple).vi"("Pathname"=w702) -> ("exists?"=w693:bool)
            n270 = And(x=w693, y=w694) -> (x .and. y?=w692:bool)
            n271 = case shown="False" w692 {
              tunnel: [w709 ""] -> w697
              tunnel: w696 -> [w705 _]
              tunnel: w695 -> [w703 _]
              frame False {
                w707 = "\r\n"
                n272 = Build Array(w703) -> (w704:string[])
                n273 = call "List_files_in_order_of_age.vi"("Files to Hide"=w704, "Folder"=w705) -> ("file names"=w706:string[])
                n274 = for {
                  shift-right: [w713] -> w710
                  shift-left: "Cannot find the VI to run. Specific Argument options are:" -> [w714]
                  tunnel: w706 -> [w715] mode=indexing
                  w712 = "  " ("Substring")
                  n275 = Concatenate Strings(w714, w712, w715, w712) -> (w713:string)
                }
                n276 = Concatenate Strings(w710, w707, "Please place one of these strings in the \"Specific Argument\" field.", w707) -> (w709:string)
              }
              frame True {
              }
            }
            n277 = Concatenate Strings(w684, w697) -> (w701:string)
          }
          frame "Wait (minutes)" {
            n278 = Unbundle By Name(w718) -> ("Specific Arguments"=w719:string)
            n279 = call "Wait_Case_Arg.vi"("Specific Argument"=w719) -> ("Error Comments"=w720:string)  [unwired: 1 in, 4 out]
          }
          frame "Send Message" {
          }
          frame "Synchronize With:" {
            n280 = local read "Current Sync Number"() -> (w728:i32)
            n281 = call "Synchronize_Prog_Arg.vi"("Execution Row"=w727) -> ("Error Comments"=w730:string, "Sync No"=w736:i32)  [unwired: 3 out]
            n282 = Equal?(x=w736, y=w728) -> (x = y?=w735:bool)
            n283 = Format Into String(format string="This should be Synchroisation number %d.\n" ("Format String"), w728) -> (resulting string=w733:string)  [unwired: 2 in, 1 out]
            n284 = Select(t="", s=w735, f=w733) -> (s? t:f=w731:string)
            n285 = Concatenate Strings(w731, w730) -> (w729:string)
          }
          frame "Fall Back to this Row" {
          }
          frame "Turn Off Row Repeating" {
          }
          frame "Blank Row" {
            n286 = Unbundle By Name(w749) -> ("Comments"=w755:string)
            n287 = Match Pattern(string=w755, regular expression="(No Match Info)") -> (before substring=w748:string, after substring=w752:string)  [unwired: 3 out]
            n288 = Empty String/Path?(string/path=w752) -> (empty?=w753:bool)
            n289 = Bundle By Name(cluster=w749, "Comments"=w748) -> (w747:T1)
            n290 = Select(t=w752, s=w753, f="The Row Type Selector \"%s\" was not matched. Please select the desired type.\n") -> (s? t:f=w751:string)
          }
        }
        "Checks" <- w420
        n291 = Concatenate Strings(w423, w424) -> (w422:string)
      }
      frame "Sort out start and end positions" {
        n292 = Unbundle By Name(w762) -> ("Start X"=w774:dbl, "Start Y"=w773:dbl, "Start Z"=w772:dbl, "End X"=w771:dbl, "End Y"=w770:dbl, "End Z"=w769:dbl, "Extra Commands"=w758:string)
        n293 = call "Which_Trav_Setup.vi"("Extra Command String"=w758) -> ("Traverse Setup"=w757:string)
        n294 = call "Rig_Pict_Display_Pref.vi"("Traverse Name"=w757) -> ("Which Axis is vertical?"=w768:enum16{"X Axis", "Y Axis", "Z Axis"})  [unwired: 7 out]
        n295 = case shown="\"Multi-Axis Profile\", Default" w763 {
          tunnel: [w814 FALSE w830 w843 FALSE] -> w777
          tunnel: [w813 FALSE w829 w842 FALSE] -> w776
          tunnel: [w812 FALSE w828 w841 FALSE] -> w775
          tunnel: w768 -> [w811 _ w827 w840 _]
          frame "Vertical Profile" {
            n296 = case shown="\"Z Axis\"" w811 {
              tunnel: [FALSE TRUE TRUE] -> w814
              tunnel: [TRUE FALSE TRUE] -> w813
              tunnel: [TRUE TRUE FALSE] -> w812
              frame "X Axis" {
              }
              frame "Y Axis" {
              }
              frame "Z Axis" {
              }
            }
          }
          frame "Auto Calibrate" {
          }
          frame "Lateral Profile" {
            n297 = case shown="\"Y Axis\"" w827 {
              tunnel: [TRUE TRUE TRUE] -> w830
              tunnel: [TRUE TRUE FALSE] -> w829
              tunnel: [FALSE FALSE TRUE] -> w828
              frame "X Axis" {
              }
              frame "Y Axis" {
              }
              frame "Z Axis" {
              }
            }
          }
          frame "Longitudinal Profile" {
            n298 = case shown="\"Y Axis\"" w840 {
              tunnel: [FALSE FALSE FALSE] -> w843
              tunnel: [TRUE TRUE TRUE] -> w842
              tunnel: [TRUE TRUE TRUE] -> w841
              frame "X Axis" {
              }
              frame "Y Axis" {
              }
              frame "Z Axis" {
              }
            }
          }
          frame "Multi-Axis Profile", Default {
          }
        }
        n299 = Build Array(w774, w773, w772) -> (w765:dbl[])
        n300 = Build Array(w771, w770, w769) -> (w764:dbl[])
        n301 = Build Array(w777, w776, w775) -> (w766:bool[])
        "Fixed Axis" <- w766
        n302 = for {
          tunnel: w766 -> [w784] mode=indexing
          tunnel: w765 -> [w783] mode=indexing
          tunnel: w764 -> [w782] mode=indexing
          shift-right: [w779] -> w761
          shift-left: w762 -> [w780]
          i -> [w781]
          n303 = case shown="True" w784 {
            tunnel: w783 -> [_ w790]
            tunnel: w782 -> [_ w789]
            tunnel: w781 -> [_ w788]
            tunnel: w780 -> [w785 w787]
            tunnel: [w785 w786] -> w779
            frame False {
            }
            frame True {
              n304 = Not A Number/Path/Refnum?(number/path/refnum=w790) -> (NaN/Path/Refnum?=w791:bool)
              n305 = Not A Number/Path/Refnum?(number/path/refnum=w789) -> (NaN/Path/Refnum?=w793:bool)
              n306 = Exclusive Or(1:w793, 2:w791) -> (0:w792:bool)
              n307 = case shown="True" w792 {
                tunnel: w791 -> [_ w801]
                tunnel: w790 -> [_ w800]
                tunnel: w789 -> [_ w799]
                tunnel: w788 -> [_ w798]
                tunnel: w787 -> [w794 w797]
                tunnel: [w794 w796] -> w786
                frame False {
                }
                frame True {
                  n308 = Select(t=w799, s=w801, f=w800) -> (s? t:f=w795:dbl)
                  n309 = case shown="2" w798 {
                    tunnel: w797 -> [w804 w807 w810]
                    tunnel: [w803 w806 w809] -> w796
                    tunnel: w795 -> [w802 w805 w808]
                    frame 0, Default {
                      n310 = Bundle By Name(cluster=w804, "Start X"=w802, "End X"=w802) -> (w803:T1)
                    }
                    frame 1 {
                      n311 = Bundle By Name(cluster=w807, "Start Y"=w805, "End Y"=w805) -> (w806:T1)
                    }
                    frame 2 {
                      n312 = Bundle By Name(cluster=w810, "Start Z"=w808, "End Z"=w808) -> (w809:T1)
                    }
                  }
                }
              }
            }
          }
        }
      }
      frame "Check for position NaNs" {
        n313 = global read "Extra_Commands_Global.vi" "Skip Traverse Position Demand"() -> (w859:string)
        n314 = Unbundle By Name(w862) -> ("Extra Commands"=w858:string, "Start X"=w871:dbl, "Start Y"=w869:dbl, "Start Z"=w870:dbl, "End X"=w868:dbl, "End Y"=w867:dbl, "End Z"=w866:dbl)
        n315 = call "Extra_Commands.vi"("String to Search"=w858, "Command"=w859) -> ("Command Found"=w856:bool)  [unwired: 1 in, 4 out]
        n316 = case shown="False" w856 {
          tunnel: w871 -> [w886 _]
          tunnel: w870 -> [w885 _]
          tunnel: w869 -> [w884 _]
          tunnel: w868 -> [w883 _]
          tunnel: w867 -> [w882 _]
          tunnel: w866 -> [w881 _]
          tunnel: [w877 w887] -> w865
          tunnel: [w876 TRUE] -> w864
          tunnel: "" -> [w875 w887]
          frame False {
            n317 = Build Array(w886, w884, w885, w883, w882, w881) -> (w880:dbl[])
            n318 = Not A Number/Path/Refnum?(number/path/refnum=w880) -> (NaN/Path/Refnum?=w879:bool[])
            n319 = Or Array Elements(Boolean array=w879) -> (logical OR=w876:bool)
            n320 = Select(t="Some of the Start and End positions are NaN.\n" ("f"), s=w876, f=w875) -> (s? t:f=w877:string)
          }
          frame True {
          }
        }
        n321 = case shown="\"Set Tunnel Speed Only\", Default" w860 {
          tunnel: w864 -> [_ w893]
          tunnel: ["Check source details" ("t") w892] -> w863
          frame "Multi-Axis Profile" {
          }
          frame "Set Tunnel Speed Only", Default {
            n322 = Select(t="Check source details", s=w893, f="Check profile rows") -> (s? t:f=w892:string)
          }
        }
        n323 = Concatenate Strings(w873, w865) -> (w872:string)
      }
      frame "Check for Start NaNs" {
        n324 = Unbundle By Name(w899) -> ("Extra Commands"=w895:string, "Start X"=w904:dbl, "Start Y"=w902:dbl, "Start Z"=w903:dbl)
        n325 = global read "Extra_Commands_Global.vi" "Skip Traverse Position Demand"() -> (w896:string)
        n326 = call "Extra_Commands.vi"("String to Search"=w895, "Command"=w896) -> ("Command Found"=w894:bool)  [unwired: 1 in, 4 out]
        n327 = case shown="True" w894 {
          tunnel: w904 -> [w916 _]
          tunnel: w903 -> [w915 _]
          tunnel: w902 -> [w914 _]
          tunnel: "" -> [w911 w917]
          tunnel: [w909 w917] -> w900
          frame False {
            n328 = Build Array(w916, w914, w915) -> (w913:dbl[])
            n329 = Not A Number/Path/Refnum?(number/path/refnum=w913) -> (NaN/Path/Refnum?=w912:bool[])
            n330 = Or Array Elements(Boolean array=w912) -> (logical OR=w908:bool)
            n331 = Select(t="Some of the Start coordinates are NaN.\n" ("f"), s=w908, f=w911) -> (s? t:f=w909:string)
          }
          frame True {
          }
        }
        n332 = Concatenate Strings(w906, w900) -> (w905:string)
      }
      frame "Check profile rows" {
        n333 = call "Create_Pos_array.vi"("Traverse line"=w927) -> ("Traverse line Out"=w926:T1, "Error Messages"=w925:string)  [unwired: 7 out]
        n334 = Unbundle By Name(w927) -> ("Start X"=w949:dbl, "Start Y"=w948:dbl, "Start Z"=w947:dbl, "End X"=w946:dbl, "End Y"=w945:dbl, "End Z"=w944:dbl, "Specific Arguments"=w938:string, "Spacing"=w933:T2, "No. of pts."=w932:i32)
        n335 = local read "Fixed Axis"() -> (w931:bool[])
        n336 = Build Array(w949, w948, w947) -> (w929:dbl[])
        n337 = Build Array(w946, w945, w944) -> (w930:dbl[])
        n338 = case shown="\"Linear\"" w933 {
          tunnel: w938 -> [_ _ _ _ w984]
          tunnel: ["" w957 "\"N/A\" is not a valid point spacing.\n" "" w979] -> w937
          tunnel: w932 -> [_ _ _ _ w983]
          tunnel: w931 -> [_ w955 _ _ _]
          tunnel: w930 -> [_ w962 _ _ _]
          tunnel: w929 -> [_ w961 _ _ _]
          frame "Linear" {
          }
          frame "Log" {
            n339 = for {
              tunnel: w962 -> [w966] mode=indexing
              tunnel: w961 -> [w965] mode=indexing
              tunnel: [w964] -> w960 mode=indexing
              tunnel: w955 -> [w963] mode=indexing
              n340 = case shown="False" w963 {
                tunnel: w966 -> [w972 _]
                tunnel: w965 -> [w971 _]
                tunnel: [w967 FALSE] -> w964
                frame False {
                  w970 = 0.001 ("y")
                  n341 = Less?(x=w972, y=w970) -> (x < y?=w968:bool)
                  n342 = Less?(x=w971, y=w970) -> (x < y?=w969:bool)
                  n343 = Or(x=w968, y=w969) -> (x .or. y?=w967:bool)
                }
                frame True {
                }
              }
            }
            n344 = Or Array Elements(Boolean array=w960) -> (logical OR=w959:bool)
            n345 = Select(t="For log spacing, Start & End positions must be greater than 0.0001.", s=w959, f="") -> (s? t:f=w957:string)
          }
          frame "N/A" {
          }
          frame "Gauss" {
          }
          frame "Specified" {
            n346 = call "Get_array_values_fr_String.vi"("String Value"=w984) -> ("Numeric Array"=w978:dbl[])  [unwired: 1 out]
            n347 = Array Size(array=w978) -> (size(s)=w977:i32)
            n348 = Decrement(x=w977) -> (x-1=w976:i32)
            n349 = Equal?(x=w976, y=w983) -> (x = y?=w982:bool)
            n350 = Select(t="", s=w982, f="The No of points and No of Arguments do not match.\n") -> (s? t:f=w979:string)
          }
        }
        n351 = for {
          tunnel: w931 -> [w990] mode=indexing
          tunnel: w929 -> [w989] mode=indexing
          tunnel: w930 -> [w988] mode=indexing
          tunnel: [w987] -> w943 mode=indexing
          shift-right: [w985] -> w922
          shift-left: bool[] [] -> [w986]
          n352 = case shown="False" w990 {
            tunnel: w989 -> [w994 w1000]
            tunnel: w988 -> [w995 w999]
            tunnel: [TRUE w998] -> w987
            tunnel: w986 -> [w992 w997]
            tunnel: [w991 w997] -> w985
            frame False {
              n353 = Not Equal?(x=w994, y=w995) -> (x != y?=w993:bool)
              n354 = Build Array (concatenate)(w992, w993) -> (w991:bool[])
            }
            frame True {
              n355 = Equal?(x=w1000, y=w999) -> (x = y?=w998:bool)
            }
          }
        }
        n356 = Array Size(array=w922) -> (size(s)=w921:i32)
        n357 = And Array Elements(Boolean array=w943) -> (logical AND=w942:bool)
        n358 = Or Array Elements(Boolean array=w922) -> (logical OR=w919:bool)
        n359 = Not Equal To 0?(x=w921) -> (x != 0?=w920:bool)
        n360 = And(x=w919, y=w920) -> (x .and. y?=w918:bool)
        n361 = Select(t="", s=w942, f="This profile moves more than one axis.\n") -> (s? t:f=w939:string)
        n362 = Select(t="", s=w918, f="The start and end points are the same for this profile.\n") -> (s? t:f=w935:string)
        n363 = Concatenate Strings(w925, w935, w939, w937) -> (w952:string)
        n364 = Concatenate Strings(w951, w952) -> (w950:string)
      }
      frame "Check source details" {
        n365 = Unbundle By Name(w1012) -> ("Emission Rate (l/min)"=w1014:dbl, "Density Ratio"=w1004:string)  [unwired: 1 out]
        n366 = Empty String/Path?(string/path=w1004) -> (empty?=w1005:bool)
        n367 = Equal?(x=w1004, y="---------" ("f")) -> (x = y?=w1003:bool)
        n368 = Or(x=w1005, y=w1003) -> (x .or. y?=w1002:bool)
        n369 = Greater Than 0?(x=w1014) -> (x > 0?=w1009:bool)
        n370 = And(x=w1009, y=w1002) -> (x .and. y?=w1013:bool)
        n371 = case shown="False" w1013 {
          tunnel: w1012 -> [w1017 w1020]
          tunnel: [w1017 w1018] -> w1011
          frame False {
          }
          frame True {
            (unwired) "The Density Ratio Box should contain either:\nCarrier 1 Only\nCarrier 2 Only\nor the relative density ratio of the mixed gas with respect to air" ("f")
            n372 = Bundle By Name(cluster=w1020, "Density Ratio"="Carrier 1 Only") -> (w1018:T1)
          }
        }
        n373 = Select(t="Check source detail 2", s=w1009, f="check entered filename etc") -> (s? t:f=w1007:string)
      }
      frame "Check source detail 2" {
        n374 = Unbundle By Name(w1044) -> ("Trace Gas Concentration (%)"=w1045:dbl, "Density Ratio"=w1046:string)
        n375 = To Upper Case(1:w1046) -> (0:w1029:string)
        n376 = To Upper Case(1:"Carrier 1 Only") -> (0:w1031:string)
        n377 = To Upper Case(1:"Carrier 2 Only") -> (0:w1030:string)
        n378 = In Range and Coerce(upper limit=ext 3.01 ("hi"), x=w1045, lower limit=ext 0.0 ("lo")) -> (In Range?=w1026:bool)  [unwired: 1 out]
        n379 = Equal?(x=w1029, y=w1031) -> (x = y?=w1036:bool)
        n380 = Equal?(x=w1029, y=w1030) -> (x = y?=w1035:bool)
        n381 = Fract/Exp String To Number(string=w1029) -> (number=w1037:dbl)  [unwired: 4 out]
        n382 = In Range and Coerce(upper limit=ext 10.0 ("hi"), x=w1037, lower limit=ext 0.05 ("lo")) -> (In Range?=w1034:bool)  [unwired: 1 out]
        n383 = Compound Arithmetic op=OR(w1036, w1035, w1034) -> (w1021:bool)
        n384 = Select(t="", s=w1026, f="The Trace Gas Concentration must be within the range of 0 to 3%.\n") -> (s? t:f=w1022:string)
        n385 = Select(t="", s=w1021, f="The Density Ratio Box should contain either:\nCarrier 1 Only\nCarrier 2 Only\nor the relative density ratio of the mixed gas with respect to air") -> (s? t:f=w1023:string)
        n386 = Concatenate Strings(w1022, w1023) -> (w1047:string)
        n387 = Concatenate Strings(w1049, w1047) -> (w1048:string)
      }
      frame "check entered filename etc" {
        n388 = local read "Checks"() -> (w1062:string[])
        n389 = for {
          tunnel: w1062 -> [w1069] mode=indexing
          tunnel: [w1074] -> w1063 mode=indexing
          tunnel: w1059 -> [w1073]
          shift-right: [w1071] -> w1053
          shift-left: w1054 -> [w1072]
          tunnel: [w1070] -> w1052 mode=indexing
          n390 = case shown="\"Number:Of:Points\"" w1069 {
            tunnel: w1072 -> [w1076 w1084 w1106 w1121]
            tunnel: [w1077 w1087 w1112 w1117] -> w1074
            tunnel: w1073 -> [_ _ w1115 _]
            tunnel: [w1076 w1084 w1104 w1121] -> w1071
            tunnel: [TRUE ("cancelled") TRUE ("cancelled") w1099 TRUE ("cancelled")] -> w1070
            tunnel: w1069 -> [_ _ _ w1119]
            frame "Number:Of:Points" {
              n391 = Unbundle By Name(w1076) -> ("No. of pts."=w1079:i32)
              n392 = Greater?(x=w1079, y=0) -> (0:w1081:bool)
              n393 = Select(t="", s=w1081, f="For a profile the number of points should be more than 0.\n" ("Format String")) -> (s? t:f=w1077:string)
            }
            frame "Averaging:Time:(mins)" {
              n394 = Unbundle By Name(w1084) -> ("Averaging time (min)"=w1086:dbl)
              n395 = Greater Than 0?(x=w1086) -> (x > 0?=w1085:bool)
              n396 = Select(t="", s=w1085, f="The averaging time should be greater than zero.\n" ("Format String")) -> (s? t:f=w1087:string)
            }
            frame "Filename:HD:Users" {
              w1113 = FALSE  # Show Error handler
              n397 = Unbundle By Name(w1106) -> ("Filename"=w1090:path, "Row No"=w1101:i32, "Row Type Selector"=w1097:T3)
              n398 = call "Row_type_selector_string.vi"("Mode"=w1097) -> ("Output string"=w1096:string)
              n399 = call "Current_Filepath.vi"("Filename in"=w1090, "Data Type"="Results") -> ("Filename Out"=w1091:path)  [unwired: 1 out]
              n400 = Path To String(path=w1091) -> (string=w1110:string)
              n401 = Not A Number/Path/Refnum?(number/path/refnum=w1091) -> (NaN/Path/Refnum?=w1094:bool)
              n402 = Equal?(x=Multi_run_mode."Run VI Named:" ("Mode"), y=w1115) -> (x = y?=w1114:bool)
              n403 = Match Pattern(string=w1110, regular expression="-------" ("f")) -> (match substring=w1109:string)  [unwired: 4 out]
              n404 = Empty String/Path?(string/path=w1109) -> (empty?=w1095:bool)
              n405 = Format Into String(format string=" For Row  %d %s." ("Comment"), w1101, w1096) -> (resulting string=w1100:string)  [unwired: 2 in, 1 out]
              n406 = Compound Arithmetic op=AND(w1095, invert w1094) -> (w1093:bool)
              n407 = Select(t=w1091, s=w1093, f=path "") -> (s? t:f=w1108:path)
              n408 = call "Results_filename_checker.vi"("Filelength"=45, "Warn if Already Exists"=w1114, "Comment"=w1100, "Show Error handler"=w1113, "Results file"=w1108) -> ("Error String"=w1112:string, "cancelled"=w1103:bool, "Results file output"=w1105:path)  [unwired: 1 out]
              n409 = Bundle By Name(cluster=w1106, "Filename"=w1105) -> (w1104:T1)
              n410 = Not(x=w1103) -> (.not. x?=w1099:bool)
            }
            frame "No Match", Default {
              n411 = Concatenate Strings(w1119, " Has not been programmed.\n" ("string")) -> (w1117:string)
            }
          }
        }
        n412 = local read "Editted Row"() -> (w1056:bool)
        n413 = And Array Elements(Boolean array=w1052) -> (logical AND=w1051:bool)
        n414 = Concatenate Strings(w1063) -> (w1061:string)
        n415 = Concatenate Strings(w1060, w1061) -> (w1055:string)
        n416 = Empty String/Path?(string/path=w1055) -> (empty?=w1058:bool)
        n417 = case shown="False" w1058 {
          tunnel: ["Open Front Panel" w1067] -> w1057
          tunnel: w1056 -> [_ w1068]
          frame False {
          }
          frame True {
            n418 = Select(t="Close Front Panel", s=w1068, f="End") -> (s? t:f=w1067:string)
          }
        }
      }
      frame "Open Front Panel" {
        w1126 = TRUE  # Front Panel Window:Open
        n419 = Current VI's Path() -> (path=w1127:path)
        n420 = call "Open_Close_Front_Panel.ph.vi"("Front Panel Window:Open"=w1126, "VI path"=w1127) -> ()  [unwired: 2 out]
        n421 = local write "Editted Row"(TRUE ("Editted Row")) -> ()
        n422 = local write "Execution Row"(w1123) -> ()
      }
      frame "What to do next?" {
        w1137 = ""
        w1135 = "[\r\n]"
        n423 = local read "Execution Row"() -> (w1133:T1)
        n424 = Wait Until Next ms Multiple(millisecond multiple=u32 100) -> ()  [unwired: 1 out]
        n425 = Unbundle By Name(w1133) -> ("Row Type Selector"=w1149:T3, "Specific Arguments"=w1144:string, "Extra Commands"=w1142:string, "Density Ratio"=w1136:string)
        n426 = Not Equal?(x=Multi_run_mode."Blank Row" ("Mode"), y=w1149) -> (x != y?=w1145:bool)
        n427 = call "Replace_Character.vi"("Replace with"=w1137, "Input String"=w1144, "Search For"=w1135) -> ("Output string"=w1143:string)  [unwired: 1 out]
        n428 = call "Replace_Character.vi"("Replace with"=w1137, "Input String"=w1142, "Search For"=w1135) -> ("Output string"=w1141:string)  [unwired: 1 out]
        n429 = call "Replace_Character.vi"("Replace with"=w1137, "Input String"=w1136, "Search For"=w1135) -> ("Output string"=w1134:string)  [unwired: 1 out]
        n430 = Compound Arithmetic op=OR("Edit in Excel", "OK") -> (w1146:bool)
        n431 = Bundle By Name(cluster=w1133, "Specific Arguments"=w1143, "Extra Commands"=w1141, "Density Ratio"=w1134) -> (w1131:T1)
        n432 = Compound Arithmetic op=AND(w1146, w1145) -> (w1139:bool)
        n433 = Not Equal?(x=w1131, y=w1133) -> (x != y?=w1132:bool)
        n434 = Not(x="Edit in Excel") -> (.not. x?=w1130:bool)
        n435 = case shown="True" w1132 {
          tunnel: w1131 -> [_ w1153]
          frame False {
          }
          frame True {
            n436 = local write "Execution Row"(w1153) -> ()
          }
        }
        n437 = case shown="True" w1130 {
          tunnel: ["Close Front Panel" w1158] -> w1138
          tunnel: w1139 -> [_ w1157]
          frame False {
          }
          frame True {
            n438 = Select(t="Clean Up Row", s=w1157, f="What to do next?") -> (s? t:f=w1158:string)
          }
        }
        "Error Comments" <- w1140
      }
      frame "Clean Up Row" {
        n439 = call "Traverse_Control_Ch_Names.vi"("Mode"=T4."All Channel Names") -> ("Channel names"=w1167:string[])  [unwired: 1 in]
        n440 = call "Trav_Cluster_to_Row.vi"("Traverse line in"=w1162, "Row Number"=w1163, "Channel names"=w1167) -> ("Traverse line Out"=w1165:T1)  [unwired: 4 out]
      }
      frame "Close Front Panel" {
        w1171 = FALSE  # Front Panel Window:Open
        n441 = Current VI's Path() -> (path=w1172:path)
        n442 = call "Open_Close_Front_Panel.ph.vi"("Front Panel Window:Open"=w1171, "VI path"=w1172) -> ()  [unwired: 2 out]
      }
      frame "End" {
        n443 = local read "Editted Row"() -> (w1180:bool)
        n444 = case shown="True" w1180 {
          tunnel: w1179 -> [w1183 w1186]
          tunnel: [w1183 w1185] -> w1177
          tunnel: w1178 -> [_ w1184]
          frame False {
          }
          frame True {
            n445 = call "Traverse_Control_Ch_Names.vi"("Mode"=T4."All Channel Names") -> ("Channel names"=w1187:string[])  [unwired: 1 in]
            n446 = call "Trav_Cluster_to_Row.vi"("Traverse line in"=w1186, "Row Number"=w1184, "Channel names"=w1187) -> ("Traverse line Out"=w1185:T1)  [unwired: 4 out]
          }
        }
        n447 = local write "Error Comments"(w1181) -> ()
      }
    }
    "Traverse line Out" <- w8
  }
  "Execution Row Out" <- w2
  "Continue?" <- w1
